vi "Cryo-Con Get Loop Type.vi"(8 "error in (no error)":errorcluster, 10 "Loop number":i32=1, 11 "VISA Resource Name":refnum<visa-resource-name>) -> (0 "error out":errorcluster, 2 "Set T":T1=enum."Manual", 3 "VISA Resource Name Out":refnum<visa-resource-name>)   [LabVIEW 2021]
uses:
  Temperature Controller/Controls/Control Mode.ctl
  GPIB/VISA  Send Receive.vi
  Simple VISA Reader/Simple VISA Reader Driver.lvclass
panel:
  out "data string out":string
  out "output string":string
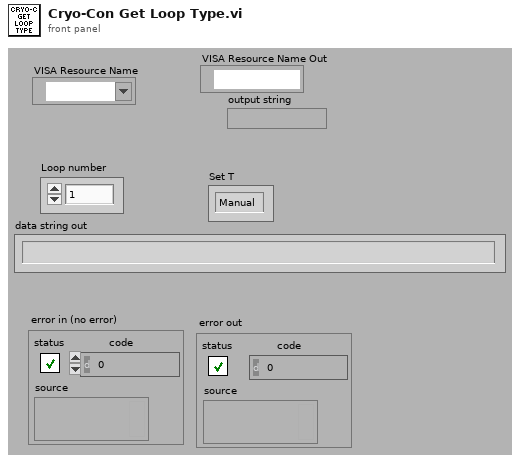
[diagram p1: front panel]
types:
  T1 = typedef "Control Mode.ctl" = enum16{"Off", "PID", "Ramp", "Manual", "Table"}
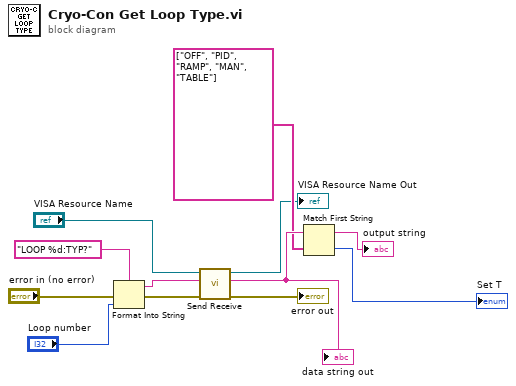
[diagram p0: block diagram]
diagram:
  n1 = Format Into String(format string="LOOP %d:TYP?", error in="error in (no error)", "Loop number") -> (resulting string=w3:string, error out=w2:errorcluster)  [unwired: 1 in]
  n2 = call-poly "Send Receive.vi"("error in (no error)"=w2, "data string in"=w3, "VISA Resource Name"="VISA Resource Name") -> ("error out"=→"error out":errorcluster, "data string out"=w11:string, "VISA Resource Name Out"=→"VISA Resource Name Out":refnum<visa-resource-name>)  [unwired: 6 in]
  "data string out" <- w11
  n3 = Match First String(2:string[] ["OFF", "PID", "RAMP", "MAN", "TABLE"] ("string array"), 3:w11) -> (0:→"Set T":i32, 1:→"output string":string)
